vi "FTW-ERR-ThrowConditionalError.vi"(7 "Error Message":string, 9 "Error Code":i32, 11 "error in":errorcluster, 12 "Throw Error?":bool, 13 "Source Level":i32 caption="Source Level (0 = This VI's caller)") -> (15 "error out":errorcluster)   [LabVIEW 2018]
doc: "Throws an error if the \"Error Code\" input is non-zero."
panel:
  # "Inputs"
  # "Outputs"
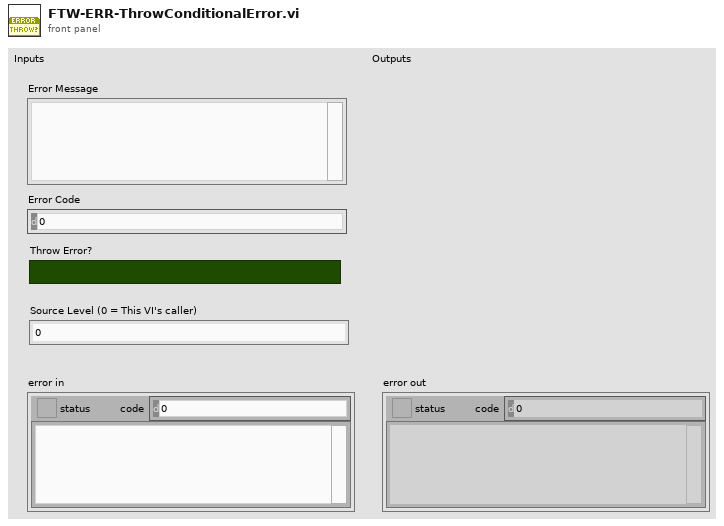
[diagram p1: front panel]
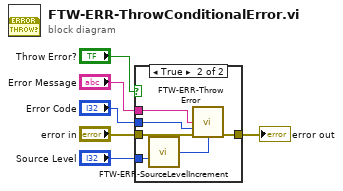
[diagram p0: block diagram]
diagram:
  n1 = case shown="True" "Throw Error?" {
    tunnel: "error in" -> [w7 w12]
    tunnel: [w7 w13] -> w5
    tunnel: "Error Message" -> [_ w11]
    tunnel: "Error Code" -> [_ w10]
    tunnel: "Source Level" -> [_ w9]
    frame False {
    }
    frame True {
      n2 = call "FTW-ERR-SourceLevelIncrement.vi"("SourceLevelIn"=w9) -> ("SourceLevelOut"=w8:i32)
      n3 = call "FTW-ERR-ThrowError.vi"("Error Message"=w11, "Error Code"=w10, "error in"=w12, "Source Level"=w8) -> ("error out"=w13:errorcluster)  [unwired: 11 in]
    }
  }
  "error out" <- w5
